vi "Get Scanner.vi"(8 "error in (no error)":errorcluster, 11 "Microwave in":refnum<class "Microwave.lvclass">) -> (0 "error out":errorcluster, 2 "Default Scanner out":refnum<class "Scanner.lvclass">)   [LabVIEW 2012, in "Microwave.lvclass"]
doc: "(Dynamic) Returns the default Scanner object that scans over this Scannable. (Note that a Scannable may have multiple Scanners associated with it.) A Scanner is an analogue to an Iterator class in other languages."
uses:
  Microwave.lvclass
  Scanners/Scanner/Scanner.lvclass
  Utility Classes/Scannable/Scannable.lvclass
  Scanners/Microwave Freq Scan/Microwave Freq Scan.lvclass
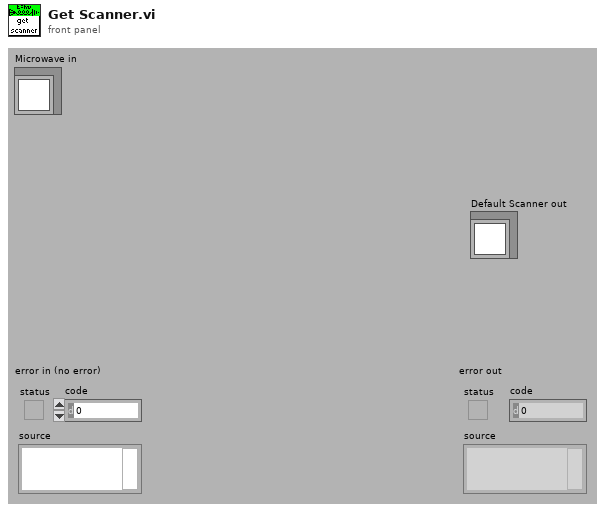
[diagram p1: front panel]
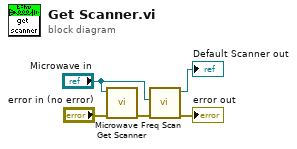
[diagram p0: block diagram]
diagram:
  n1 = call-parent "Get Scanner.vi"("error in (no error)"="error in (no error)", "Scannable in"="Microwave in") -> ("error out"=w2:errorcluster)  [unwired: 9 out]
  n2 = call "Microwave Freq Scan.vi"("error in (no error)"=w2, "Microwave.lvclass"="Microwave in") -> ("error out"=→"error out":errorcluster, "Microwave Freq Scan out"=→"Default Scanner out":refnum<class "Microwave Freq Scan.lvclass">)  [unwired: 8 out]
